vi "输入中心坐标画矩形.vi"(0 "Image In":T2, 1 "Color":u32(colorbox)=16711680, 2 "中心坐标":cluster{"P_X":i32, "P_Y":i32}, 3 "W":i32, 5 "H":i32, 8 "画框?":bool) -> (4 "ROI Descriptor":T1 {"Contours"."Type" items=["No Selection", "Point", "Line", "Rectangle", "Oval", "Polygon", "Freehand Region", "Annulus", "Unused2", "Unused3", "Broken Line", "Freehand Line", "Rotated Rectangle"]}, 6 "Image Out":T2, 7 "矩形框":dbl[](array[numeric]))   [LabVIEW 2014]
uses:
  <vilib>/vision/Image Controls.llb/IMAQ Image.ctl
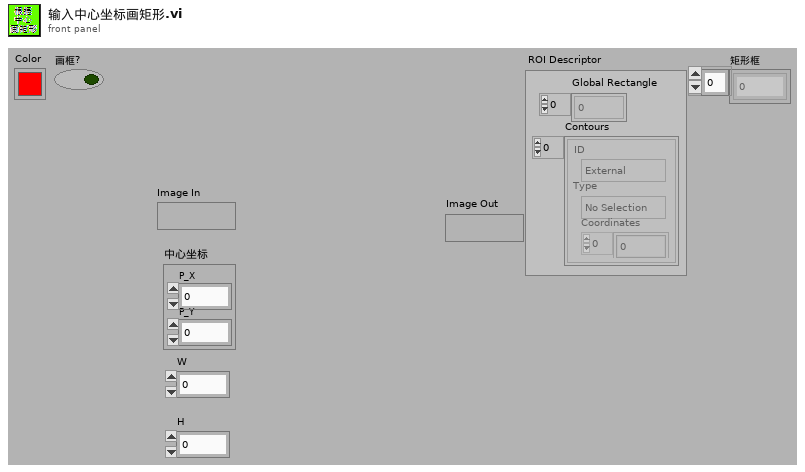
[diagram p1: front panel]
types:
  T1 = typedef "ROI Descriptor" = cluster{"Global Rectangle":i32[], "Contours":cluster{"ID":enum32{"External", "Internal"}, "Type":u32, "Coordinates":i32[]}[]}
  T2 = typedef "IMAQ Image.ctl" = refnum<image>
  T3 = cluster{"[0]":dbl, "[1]":dbl, "[2]":dbl, "[3]":dbl}
  T4 = cluster{"[0]":dbl, "[1]":dbl, "[2]":dbl, "[3]":dbl, "[4]":dbl}
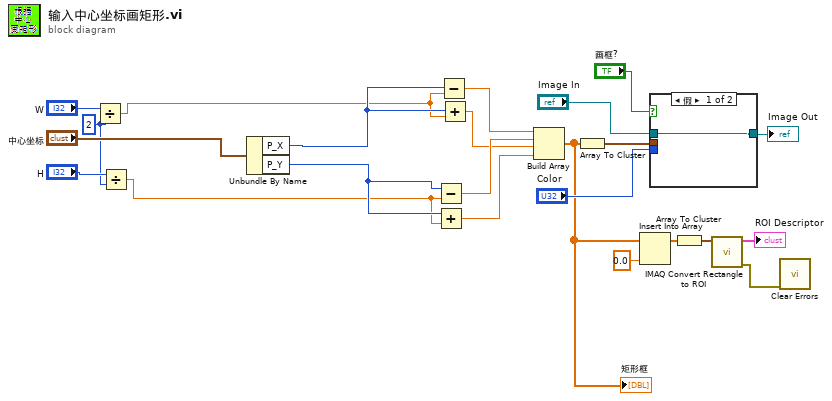
[diagram p0: block diagram]
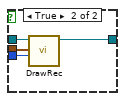
[diagram p2: hidden frame]
diagram:
  w8 = 2 ("y")
  n1 = Divide(x="W", y=w8) -> (x/y=w19:dbl)
  n2 = Divide(x="H", y=w8) -> (x/y=w17:dbl)
  n3 = Unbundle By Name("中心坐标") -> ("P_X"=w21:i32, "P_Y"=w22:i32)
  n4 = Subtract(x=w22, y=w17) -> (x-y=w15:dbl)
  n5 = Add(x=w22, y=w17) -> (x+y=w13:dbl)
  n6 = Subtract(x=w21, y=w19) -> (x-y=w16:dbl)
  n7 = Add(x=w21, y=w19) -> (x+y=w14:dbl)
  n8 = Build Array(w16, w15, w14, w13) -> (w7:dbl[])
  "矩形框" <- w7
  n9 = Array To Cluster(array=w7) -> (cluster=w12:T3)
  n10 = Insert Into Array(array=w7, new element=0.0 ("新元素/子数组")) -> (w5:dbl[])  [unwired: 1 in]
  n11 = case shown="假" "画框?" {
    tunnel: w12 -> [_ w28]
    tunnel: "Image In" -> [w24 w27]
    tunnel: "Color" -> [_ w26]
    tunnel: [w24 w25] -> w9
    frame False {
    }
    frame True {
      n12 = call "DrawRec.vi"("Color"=w26, "Rectangle"=w28, "Image"=w27) -> ("Image Out"=w25:T2)  [unwired: 8 in]
    }
  }
  "Image Out" <- w9
  n13 = Array To Cluster(array=w5) -> (cluster=w4:T4)
  n14 = call "IMAQ Convert Rectangle to ROI"("Rectangle"=w4) -> ("error out"=w2:errorcluster, "ROI Descriptor"=→"ROI Descriptor":T1)  [unwired: 8 in]
  n15 = call <vilib>:"Clear Errors.vi"("error in (no error)"=w2) -> ()  [unwired: 5 in, 2 out]
